vi "Intan_Serial_Close.vi"() -> ()   [LabVIEW 2017]
panel:
  out "error out":errorcluster
  in  "VISA resource name":refnum<visa-resource-name>="COM1"
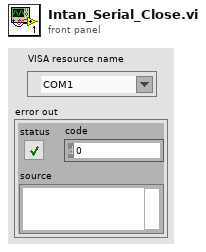
[diagram p1: front panel]
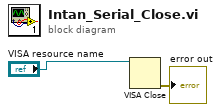
[diagram p0: block diagram]
diagram:
  n1 = VISA Close(VISA resource name="VISA resource name") -> (error out=→"error out":errorcluster)  [unwired: 1 in]
